vi "HTSResistance.vi"() -> ()   [LabVIEW 2017]
uses:
  <vilib>/Analysis/6fits.llb/Curve Fitting Criteria.ctl
  Keysight N8731A conversion/Keysight N8900 Series.lvlib
  <vilib>/Analysis/NI_AALPro.lvlib
panel:
  out "Averaged resistance":dbl
  in  "Measurements":i32=1
  in  "filename":string caption="Discard data if empty"
  out "Resistance (latest)":dbl
  out "V(I)":T1(graph)
  out "Time Data":dbl[](array[numeric])
  out "Voltage Data":dbl[](array[numeric])
  out "Current Data":dbl[](array[numeric])
  out "I(t)":T1(graph)
  out "start time":dbl format="%_19f"
  in  "Points":dbl=500.0
  in  "OV Value (10V)":dbl=10.0
  in  "VISA resource name":refnum<visa-resource-name>
  in  "Keithley (1)/PSU (0)":bool=TRUE caption="Voltage Source"
  in  "Voltage limit [V]":dbl
  in  "Current limit [A]":dbl
  in  "Time between measurements [ms]":dbl=250.0
  # "Program will set Voltage and Current to specified limits, then make\nmeasurements at specified intervals until the measurement is either\nmanually stopped or measurement time runs out. Once the\nmeasurement is over, Resistance and inductance are calculated, and\nthe coil is run down in two steps."
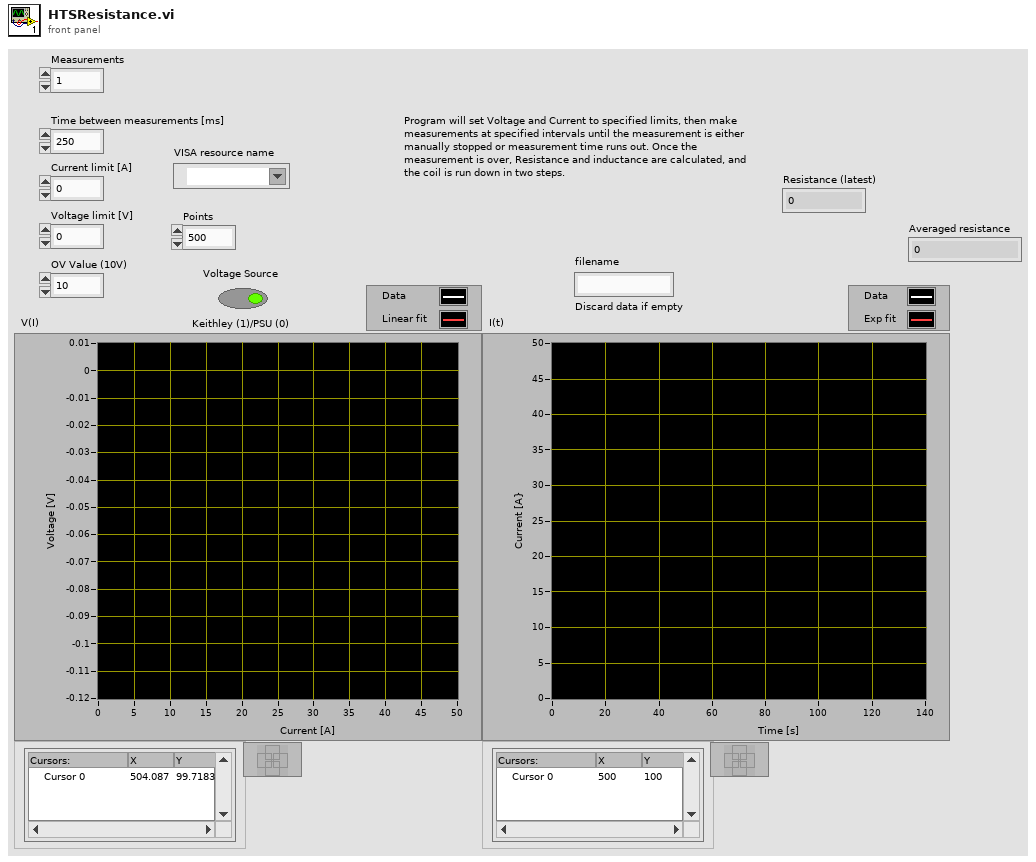
[diagram p1: front panel]
types:
  T1 = cluster{"Current Data":dbl[], "Best Linear Fit":dbl[]}[]
  T2 = typedef "NI_AALPro.lvlib/Curve Fitting Criteria.ctl" = u16
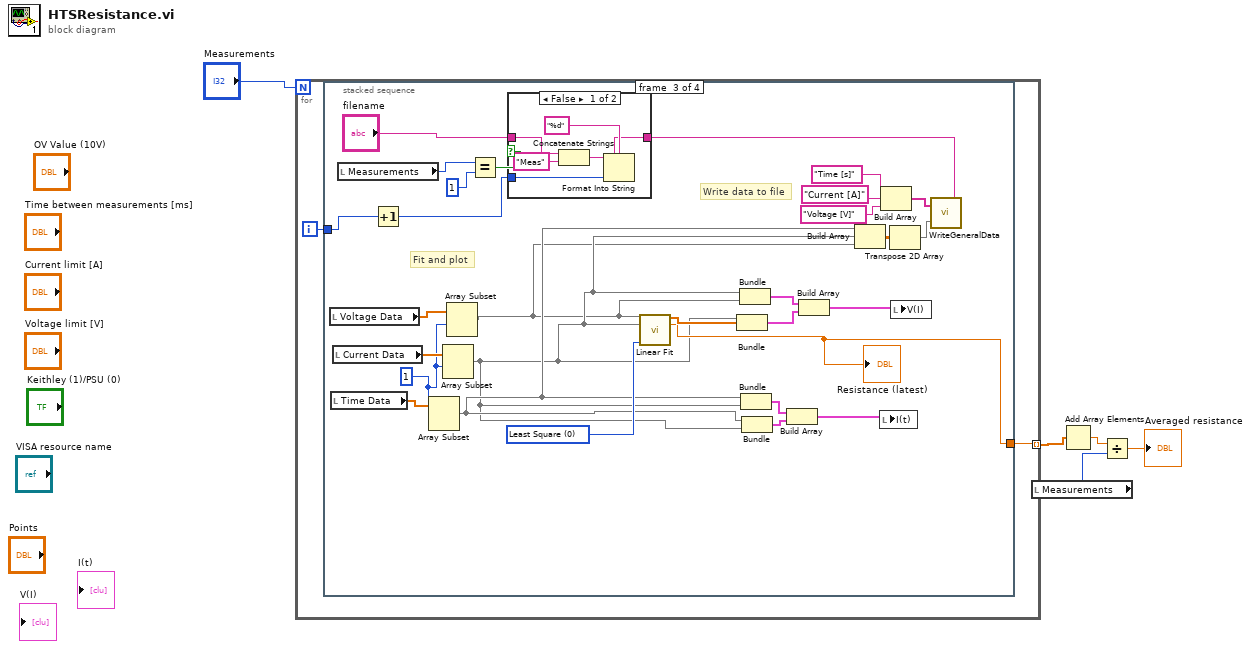
[diagram p0: block diagram]
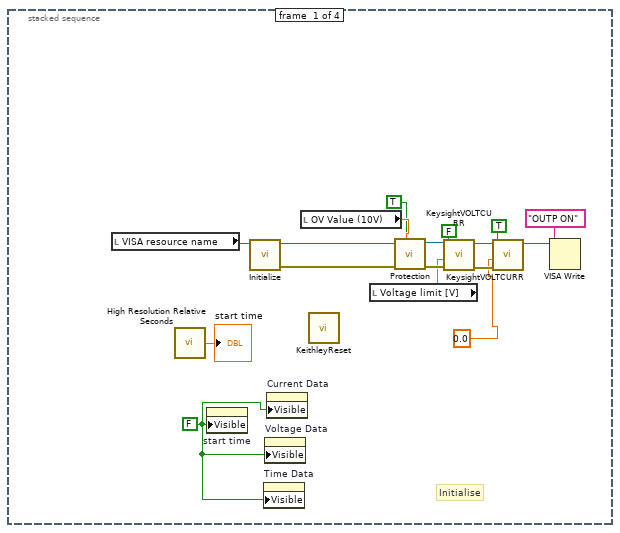
[diagram p2: hidden frame]
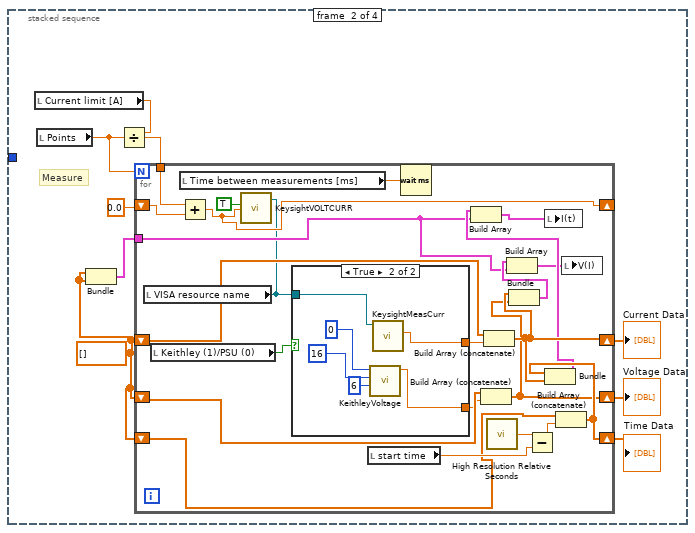
[diagram p3: hidden frame]
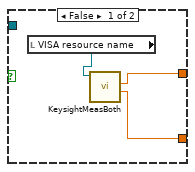
[diagram p4: hidden frame]
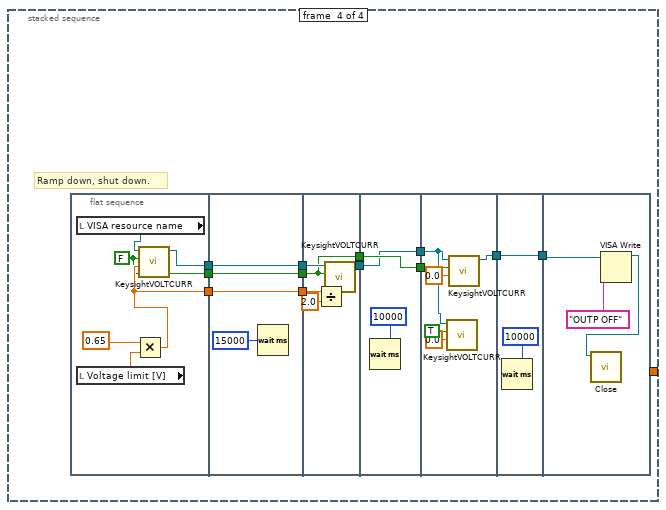
[diagram p6: hidden frame]
diagram:
  n1 = for {
    N: "Measurements" -> [_]
    tunnel: [w7] -> w3 mode=indexing
    i -> [w6]
    n2 = stacked-sequence {
      tunnel: [_ _ w86 _] -> w7
      tunnel: w6 -> [_ _ w67 _]
      frame #0 {
        w11 = FALSE ("Visible")
        # "Initialise"
        n3 = local read "VISA resource name"() -> (w22:refnum<visa-resource-name>)
        n4 = call <vilib>:"High Resolution Relative Seconds.vi"() -> ("relative seconds"=→"start time":dbl)
        n5 = property on="start time" class="DigNum (strict)"("Visible"=w11) -> ()  [unwired: 2 in, 2 out]
        n6 = call "Initialize.vi"("VISA resource name"=w22) -> ("error out"=w24:errorcluster, "VISA resource name out"=w23:refnum<visa-resource-name>)  [unwired: 9 in]
        n7 = property on="Time Data" class="Arr (strict)"("Visible"=w11) -> ()  [unwired: 2 in, 2 out]
        n8 = property on="Voltage Data" class="Arr (strict)"("Visible"=w11) -> ()  [unwired: 2 in, 2 out]
        n9 = property on="Current Data" class="Arr (strict)"("Visible"=w11) -> ()  [unwired: 2 in, 2 out]
        n10 = local read "OV Value (10V)"() -> (w21:dbl)
        n11 = call "KeithleyReset.vi"() -> ()  [unwired: 11 in, 1 out]
        n12 = local read "Voltage limit [V]"() -> (w13:dbl)
        n13 = call "Protection.vi"("OV protection"=TRUE, "error in (no error)"=w24, "OV Value (10V)"=w21, "VISA resource name"=w23) -> ("error out"=w18:errorcluster, "VISA resource name out"=w19:refnum<visa-resource-name>)  [unwired: 6 in]
        n14 = call "KeysightVOLTCURR.vi"("error in (no error)"=w18, "CURR/VOLT (A/V)"=w13, "CURR (1)/VOLT (0)"=FALSE, "VISA resource name"=w19) -> ("error out"=w15:errorcluster, "VISA resource name out"=w16:refnum<visa-resource-name>)  [unwired: 6 in]
        n15 = call "KeysightVOLTCURR.vi"("error in (no error)"=w15, "CURR/VOLT (A/V)"=0.0, "CURR (1)/VOLT (0)"=TRUE, "VISA resource name"=w16) -> ("VISA resource name out"=w10:refnum<visa-resource-name>)  [unwired: 6 in, 1 out]
        n16 = VISA Write(VISA resource name=w10, write buffer="OUTP ON") -> ()  [unwired: 1 in, 3 out]
      }
      frame #1 {
        w30 = dbl[] []
        # "Measure"
        n17 = local read "Current limit [A]"() -> (w28:dbl)
        n18 = local read "Points"() -> (w27:dbl)
        n19 = Bundle(w30, w30) -> (w29:cluster{dbl[], dbl[]})  [unwired: 1 in]
        n20 = Divide(x=w28, y=w27) -> (x/y=w25:dbl)
        n21 = for {
          N: w27 -> [_]
          shift-right: [w45] -> w33
          shift-left: w30 -> [w53]
          shift-right: [w44] -> w32
          shift-left: w30 -> [w54]
          shift-right: [w46] -> w31
          shift-left: w30 -> [w47]
          tunnel: w29 -> [w41]
          shift-right: [w35] -> _
          shift-left: 0.0 -> [w38]
          tunnel: w25 -> [w37]
          n22 = local read "VISA resource name"() -> (w34:refnum<visa-resource-name>)
          n23 = local read "Keithley (1)/PSU (0)"() -> (w55:bool)
          n24 = local read "Time between measurements [ms]"() -> (w56:dbl)
          n25 = Add(x=w37, y=w38) -> (x+y=w35:dbl)
          n26 = call "KeysightVOLTCURR.vi"("CURR/VOLT (A/V)"=w35, "CURR (1)/VOLT (0)"=TRUE, "VISA resource name"=w34) -> ()  [unwired: 7 in, 2 out]
          n27 = case shown="True" w55 {
            tunnel: [w58 w65] -> w52
            tunnel: [w57 w64] -> w51
            tunnel: w34 -> [_ w60]
            frame False {
              n28 = local read "VISA resource name"() -> (w59:refnum<visa-resource-name>)
              n29 = call "KeysightMeasBoth.vi"("VISA resource name"=w59) -> ("VOLT"=w57:dbl, "CURR"=w58:dbl)  [unwired: 7 in, 2 out]
            }
            frame True {
              n30 = call "KeithleyVoltage.vi"("channel (6)"=6, "address (16)"=i16 16, "bus"=0) -> ("Voltage"=w64:dbl)  [unwired: 7 in, 1 out]
              n31 = call "KeysightMeasCurr.vi"("VISA resource name"=w60) -> ("CURR"=w65:dbl)  [unwired: 8 in, 2 out]
            }
          }
          n32 = local read "start time"() -> (w49:dbl)
          n33 = Wait (ms)(milliseconds to wait=w56) -> ()  [unwired: 1 out]
          n34 = Build Array (concatenate)(w54, w51) -> (w44:dbl[])
          n35 = Build Array (concatenate)(w53, w52) -> (w45:dbl[])
          n36 = call <vilib>:"High Resolution Relative Seconds.vi"() -> ("relative seconds"=w50:dbl)
          n37 = Bundle(w45, w44) -> (w42:cluster{dbl[], dbl[]})  [unwired: 1 in]
          n38 = Build Array(w42, w41) -> (w39:cluster{dbl[], dbl[]}[])
          n39 = Subtract(x=w50, y=w49) -> (x-y=w48:dbl)
          n40 = Build Array (concatenate)(w47, w48) -> (w46:dbl[])
          n41 = Bundle(w46, w45) -> (w43:cluster{dbl[], dbl[]})  [unwired: 1 in]
          n42 = Build Array(w43, w41) -> (w40:cluster{dbl[], dbl[]}[])
          n43 = local write "I(t)"(w40) -> ()
          n44 = local write "V(I)"(w39) -> ()
        }
        "Current Data" <- w33
        "Voltage Data" <- w32
        "Time Data" <- w31
      }
      frame #2 {
        w73 = 1 ("index")
        w94 = T2 0 items=["Least Square", "Least Absolute Residual", "Bisquare"] ("method")
        # "Write data to file"
        # "Fit and plot"
        n45 = local read "Voltage Data"() -> (w75:dbl[])
        n46 = local read "Time Data"() -> (w79:dbl[])
        n47 = local read "Current Data"() -> (w77:dbl[])
        n48 = local read "Measurements"() -> (w69:i32)
        n49 = Increment(x=w67) -> (x+1=w66:i32)
        n50 = Array Subset(array=w79, index=w73) -> (w78:dbl[])  [unwired: 1 in]
        n51 = Array Subset(array=w77, index=w73) -> (w76:dbl[])  [unwired: 1 in]
        n52 = Array Subset(array=w75, index=w73) -> (w74:dbl[])  [unwired: 1 in]
        n53 = Equal?(x=w69, y=1) -> (x = y?=w71:bool)
        n54 = case shown="False" w71 {
          tunnel: "filename" -> [w97 w101]
          tunnel: [w98 w101] -> w70
          tunnel: w66 -> [w99 _]
          frame False {
            n55 = Concatenate Strings(w97, "Meas" ("string")) -> (w95:string)
            n56 = Format Into String(format string="%d", initial string=w95, w99) -> (resulting string=w98:string)  [unwired: 1 in, 1 out]
          }
          frame True {
          }
        }
        n57 = call <vilib>:"Linear Fit.vi"("Y"=w74, "X"=w76, "method"=w94) -> ("Best Linear Fit"=w93:dbl[], "slope"=w86:dbl)  [unwired: 8 in, 3 out]
        "Resistance (latest)" <- w86
        n58 = Bundle(w76, "Best Linear Fit"=w93) -> (w90:cluster{dbl[], "Best Linear Fit":dbl[]})  [unwired: 1 in]
        n59 = Bundle(w76, w74) -> (w89:cluster{dbl[], dbl[]})  [unwired: 1 in]
        n60 = Bundle(w78, w76) -> (w92:cluster{dbl[], dbl[]})  [unwired: 1 in]
        n61 = Bundle(w78, w76) -> (w91:cluster{dbl[], dbl[]})  [unwired: 1 in]
        n62 = Build Array(w92, w91) -> (w87:cluster{dbl[], dbl[]}[])
        n63 = Build Array(w89, w90) -> (w88:cluster{dbl[], "Best Linear Fit":dbl[]}[])
        n64 = Build Array(w78, w76, w74) -> (w81:dbl[][])
        n65 = local write "I(t)"(w87) -> ()
        n66 = Build Array("Time [s]", "Current [A]", "Voltage [V]") -> (w82:string[])
        n67 = Transpose 2D Array(2D array=w81) -> (transposed array=w80:dbl[][])
        n68 = local write "V(I)"(w88) -> ()
        n69 = call "WriteGeneralData.vi"("filename (discard if empty)"=w70, "Array"=w80, "Column name array"=w82) -> ()
      }
      frame #3 {
        # "Ramp down, shut down."
        n70 = flat-sequence {
          tunnel: [w116] -> w112
          tunnel: [w115] -> w110
          tunnel: [w114] -> w108
          tunnel: [w122] -> w113
          tunnel: w112 -> [w122]
          tunnel: [w121] -> w111
          tunnel: w110 -> [w121]
          tunnel: [w120] -> w109
          tunnel: w108 -> [w120]
          tunnel: w113 -> [w129]
          tunnel: w111 -> [w127]
          tunnel: w109 -> [w125]
          tunnel: [w125] -> w106
          tunnel: [w124] -> w104
          tunnel: [w131] -> w107
          tunnel: w106 -> [w131]
          tunnel: [w130] -> w105
          tunnel: w104 -> [w130]
          tunnel: w107 -> [w138]
          tunnel: w105 -> [w135]
          tunnel: [w133] -> w103
          tunnel: w103 -> [w140]
          tunnel: [w140] -> w102
          tunnel: w102 -> [w143]
          frame #0 {
            w114 = FALSE ("CURR (1)/VOLT (0)")
            n71 = local read "VISA resource name"() -> (w119:refnum<visa-resource-name>)
            n72 = local read "Voltage limit [V]"() -> (w118:dbl)
            n73 = Multiply(x=0.65, y=w118) -> (x*y=w115:dbl)
            n74 = call "KeysightVOLTCURR.vi"("CURR/VOLT (A/V)"=w115, "CURR (1)/VOLT (0)"=w114, "VISA resource name"=w119) -> ("VISA resource name out"=w116:refnum<visa-resource-name>)  [unwired: 7 in, 1 out]
          }
          frame #1 {
            n75 = Wait (ms)(milliseconds to wait=u32 15000) -> ()  [unwired: 1 out]
          }
          frame #2 {
            n76 = Divide(x=w127, y=2.0) -> (x/y=w126:dbl)
            n77 = call "KeysightVOLTCURR.vi"("CURR/VOLT (A/V)"=w126, "CURR (1)/VOLT (0)"=w125, "VISA resource name"=w129) -> ("VISA resource name out"=w124:refnum<visa-resource-name>)  [unwired: 7 in, 1 out]
          }
          frame #3 {
            n78 = Wait (ms)(milliseconds to wait=u32 10000) -> ()  [unwired: 1 out]
          }
          frame #4 {
            n79 = call "KeysightVOLTCURR.vi"("CURR/VOLT (A/V)"=0.0, "CURR (1)/VOLT (0)"=TRUE, "VISA resource name"=w135) -> ()  [unwired: 7 in, 2 out]
            n80 = call "KeysightVOLTCURR.vi"("CURR/VOLT (A/V)"=0.0, "CURR (1)/VOLT (0)"=w138, "VISA resource name"=w135) -> ("VISA resource name out"=w133:refnum<visa-resource-name>)  [unwired: 7 in, 1 out]
          }
          frame #5 {
            n81 = Wait (ms)(milliseconds to wait=u32 10000) -> ()  [unwired: 1 out]
          }
          frame #6 {
            n82 = VISA Write(VISA resource name=w143, write buffer="OUTP OFF") -> (VISA resource name out=w141:refnum<visa-resource-name>)  [unwired: 1 in, 2 out]
            n83 = call "Close.vi"("VISA resource name"=w141) -> ()  [unwired: 10 in, 1 out]
          }
        }
      }
    }
  }
  n84 = local read "Measurements"() -> (w4:i32)
  n85 = Add Array Elements(numeric array=w3) -> (sum=w2:dbl)
  n86 = Divide(x=w2, y=w4) -> (x/y=→"Averaged resistance":dbl)
